vi "intensity_show_image.vi"() -> ()   [LabVIEW 2021]
panel:
  out "Intensity Graph 3":u8[][](graph)
  out "Intensity Graph G":u8[][](graph)
  out "Intensity Graph R":u8[][](graph)
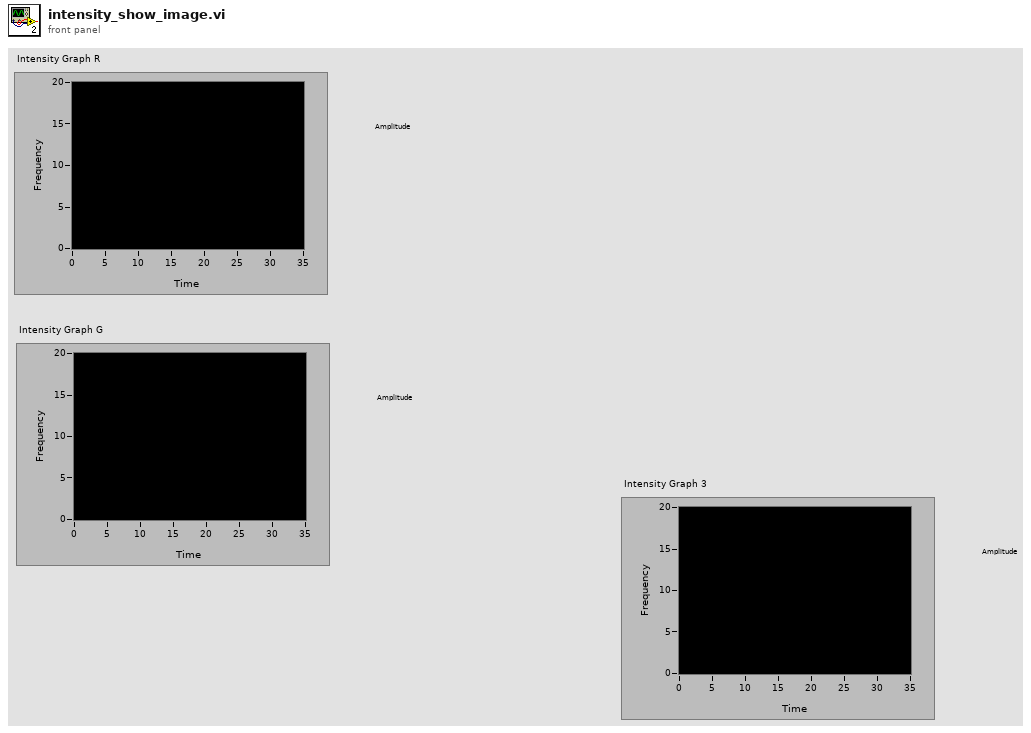
[diagram p1: front panel]
types:
  T1 = typedef "imagedata.ctl" = cluster{"image type":i32, "image depth":i32, "image":u8[], "mask":u8[], "colors":u32[], "Rectangle":cluster{"left":i16, "top":i16, "right":i16, "bottom":i16}}
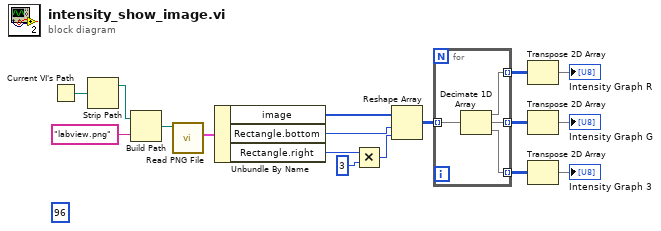
[diagram p0: block diagram]
diagram:
  (unwired) 96 ("dimension size")
  n1 = Current VI's Path() -> (path=w15:path)
  n2 = Strip Path(path=w15) -> (stripped path=w16:path)  [unwired: 1 out]
  n3 = Build Path(base path=w16, name or relative path="labview.png") -> (appended path=w14:path)
  n4 = call <vilib>:"Read PNG File.vi"("path to PNG file"=w14) -> ("image data"=w13:T1)  [unwired: 8 in, 2 out]
  n5 = Unbundle By Name(w13) -> ("image"=w12:u8[], "Rectangle.bottom"=w10:i16, "Rectangle.right"=w9:i16)
  n6 = Multiply(x=w9, y=i16 3) -> (x*y=w8:i16)
  n7 = Reshape Array(w12, w10, w8) -> (w7:u8[][])
  n8 = for {
    tunnel: w7 -> [w21] mode=indexing
    tunnel: [w20] -> w6 mode=indexing
    tunnel: [w19] -> w4 mode=indexing
    tunnel: [w18] -> w3 mode=indexing
    n9 = Decimate 1D Array(w21) -> (w20:u8[], w19:u8[], w18:u8[])
  }
  n10 = Transpose 2D Array(2D array=w6) -> (transposed array=→"Intensity Graph R":u8[][])
  n11 = Transpose 2D Array(2D array=w4) -> (transposed array=→"Intensity Graph G":u8[][])
  n12 = Transpose 2D Array(2D array=w3) -> (transposed array=→"Intensity Graph 3":u8[][])
